vi "Read Costs.vi"(11 "Blueprint in":refnum<class "Blueprint.lvclass">) -> (2 "Costs":T1, 3 "Blueprint out":refnum<class "Blueprint.lvclass">)   [LabVIEW 2021, in "d19.lvlib" / "Blueprint.lvclass"]
uses:
  Blueprint.lvclass
  Blueprint.lvclass/Blueprint.ctl
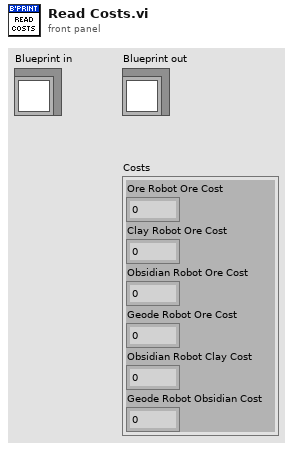
[diagram p1: front panel]
types:
  T1 = cluster{"Ore Robot Ore Cost":u8, "Clay Robot Ore Cost":u8, "Obsidian Robot Ore Cost":u8, "Geode Robot Ore Cost":u8, "Obsidian Robot Clay Cost":u8, "Geode Robot Obsidian Cost":u8}
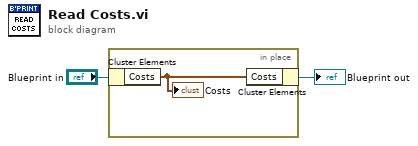
[diagram p0: block diagram]
diagram:
  n1 = in-place {
    n2 = in-place-cluster #1("Blueprint in") -> ("Costs"=w3:T1)
    "Costs" <- w3
    n3 = in-place-cluster #1("Costs"=w3) -> (→"Blueprint out":refnum<class "Blueprint.lvclass">)
  }
